vi "Main.vi"(11 "Module Admin":refnum<class "Delacor_lib_QMH_Module Admin.lvclass">) -> ()   [LabVIEW 2020, in "YP03-60CurrentSource_1.lvlib"]
doc: "This template is based off of the Queued Message Handler design pattern and the Queued Message Handler project template that ships with LabVIEW.\n\nThe main difference is that the queue is private to this module and communication between modules is performed via Broadcast and Request events.\n\nRequest events are wrapped in public API methods and are handled in the Event Handling Loop (EHL) of this VI. Any module can register for Broadcast events sent by this module. The EHL generates messages based on user interface actions.\n\nThe Message Handling Loop (MHL) processes messages generated by the EHL, or by other messages. The messages are string values, so new messages can be added easily to the Message Cases case structure in the MHL. Each message cluster can also provide an optional value for Message Data, which is a variant that can be converted to whatever message-specific data is required.\n_____\nBased on DQMH Project Template 6.0.0.91."
uses:
  YP03-60CurrentSource_1.lvlib
  <vilib>/Delacor/Delacor QMH/Libraries/Module Admin_class/Delacor_lib_QMH_Module Admin.lvclass
  CurrentSet-X Argument--cluster.ctl
  Module Data--cluster.ctl
  Stop Argument--cluster.ctl
  <vilib>/Delacor/Delacor QMH/Libraries/Message Queue_class/Delacor_lib_QMH_Message Queue.lvclass/Delacor_lib_QMH_Message Queue.ctl
  <vilib>/Delacor/Delacor QMH/Libraries/Module Admin_class/Delacor_lib_QMH_Module Admin.lvclass/Delacor_lib_QMH_Module Admin.ctl
  CurrentSet-Y Argument--cluster.ctl
  CurrentSet-Z Argument--cluster.ctl
  Output Argument--cluster.ctl
  <vilib>/Utility/miscctls.llb/LVPointTypeDef.ctl
  <vilib>/Delacor/Delacor QMH/Libraries/Message Queue_class/Delacor_lib_QMH_Enqueue Message (Single).vi
  <vilib>/Delacor/Delacor QMH/Libraries/Module Admin_class/Delacor_lib_QMH_Get External Launch.vi
  <vilib>/Utility/error.llb/Error Cluster From Error Code.vi
  <vilib>/ErrorRing/Error Ring.xnode
  <vilib>/Delacor/Delacor QMH/Libraries/Message Queue_class/Delacor_lib_QMH_Message Queue.lvclass
panel:
  in  "CurrentSet Argument":T1={"CurrentSet(A)"=0.0, "Cluster"={"VISA resource name"="COM6", "baud rate (9600)"=9600, "data bits (8)"=8, "parity (0:none)"=enum."None"}} {"Cluster"."data bits (8)" min=5 max=8 step=1; "CurrentSet(A)" min=-4.0 max=4.0 step=0.05}
  out "History:Entire Text":string="rev. 12 Tue, Feb 14, 2023 11:30:20 AM chenyu\r\n添加Request电流设置请求\n当外部调用该vi时，这个时间会被广播出去，被main函数生产结构接收到，进入从循环执行电流设置的vi\r\n"
  out "error out":errorcluster
  out "Status":string="Initial Message"
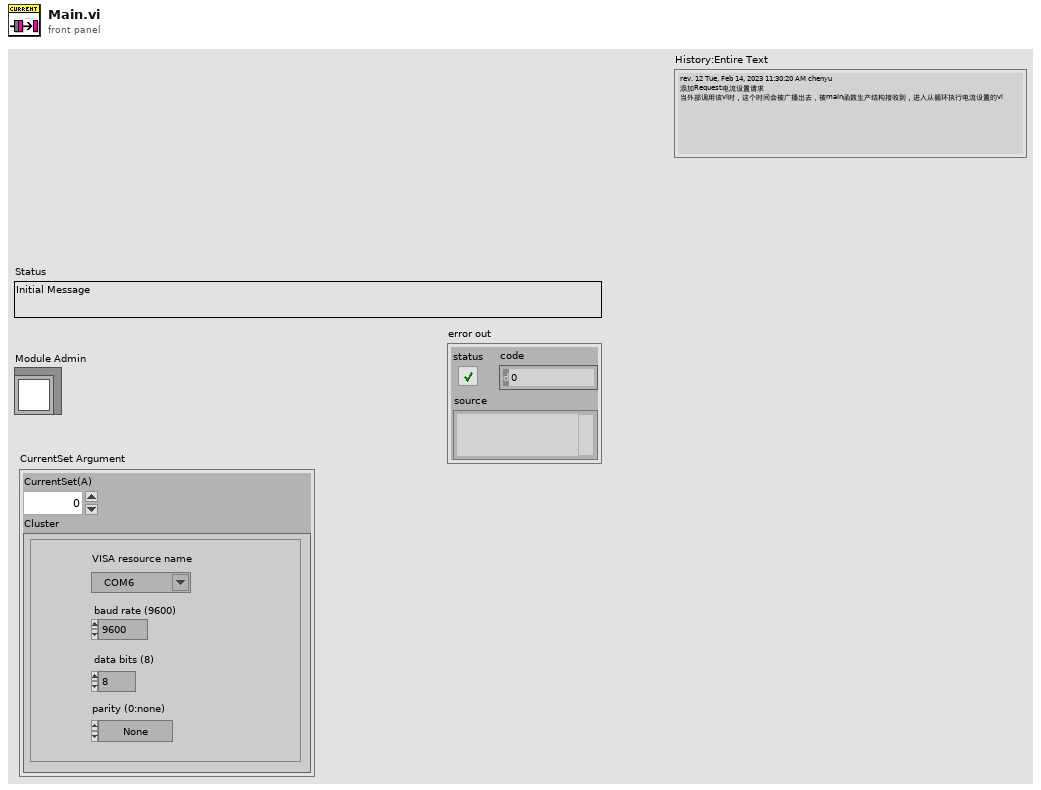
[diagram p1: front panel]
types:
  T1 = typedef "YP03-60CurrentSource_1.lvlib/CurrentSet-X Argument--cluster.ctl" = cluster{"CurrentSet(A)":dbl, "Cluster":cluster{"VISA resource name":refnum<visa-resource-name>, "baud rate (9600)":u32, "data bits (8)":u16, "parity (0:none)":enum16{"None", "Odd", "Even", "Mark", "Space"}}}
  T2 = typedef "YP03-60CurrentSource_1.lvlib/Request Events--cluster.ctl" = cluster{"Stop Module":refnum<user-event>, "Show Panel":refnum<user-event>, "Hide Panel":refnum<user-event>, "Get Module Execution Status":refnum<user-event>, "Show Diagram":refnum<user-event>, "CurrentSet-X":refnum<user-event>, "CurrentSet-Y":refnum<user-event>, "CurrentSet-Z":refnum<user-event>, "Output":refnum<user-event>}
  T3 = typedef "YP03-60CurrentSource_1.lvlib/Module Data--cluster.ctl" = cluster{"Status":string}
  T4 = enum32{"invalid lock state", "Not Locked", "Locked (No Password)", "Password-protected"}
  T5 = typedef "YP03-60CurrentSource_1.lvlib/Stop Argument--cluster.ctl" = cluster{"Origin":string, "Exit via Stop Module Req?":bool, "Wait for Module to stop?":bool}
  T6 = typedef "YP03-60CurrentSource_1.lvlib/CurrentSet-Y Argument--cluster.ctl" = cluster{"Cuurent-Y":dbl, "Cluster":cluster{"VISA resource name":refnum<visa-resource-name>, "baud rate (9600)":u32, "data bits (8)":u16, "parity (0:none)":enum16{"None", "Odd", "Even", "Mark", "Space"}}}
  T7 = typedef "YP03-60CurrentSource_1.lvlib/CurrentSet-Z Argument--cluster.ctl" = cluster{"Numeric":dbl, "Cluster":cluster{"VISA resource name":refnum<visa-resource-name>, "baud rate (9600)":u32, "data bits (8)":u16, "parity (0:none)":enum16{"None", "Odd", "Even", "Mark", "Space"}}}
  T8 = typedef "YP03-60CurrentSource_1.lvlib/Output Argument--cluster.ctl" = cluster{"Output":bool}
  T9 = typedef "LVPointTypeDef.ctl" = cluster{"Horizontal":i16, "Vertical":i16}
  T10 = enum32{"Invalid", "Standard", "Closed", "Hidden", "Minimized", "Maximized"}
  T11 = cluster{"VISA resource name":refnum<visa-resource-name>, "baud rate (9600)":u32, "data bits (8)":u16, "parity (0:none)":enum16{"None", "Odd", "Even", "Mark", "Space"}}
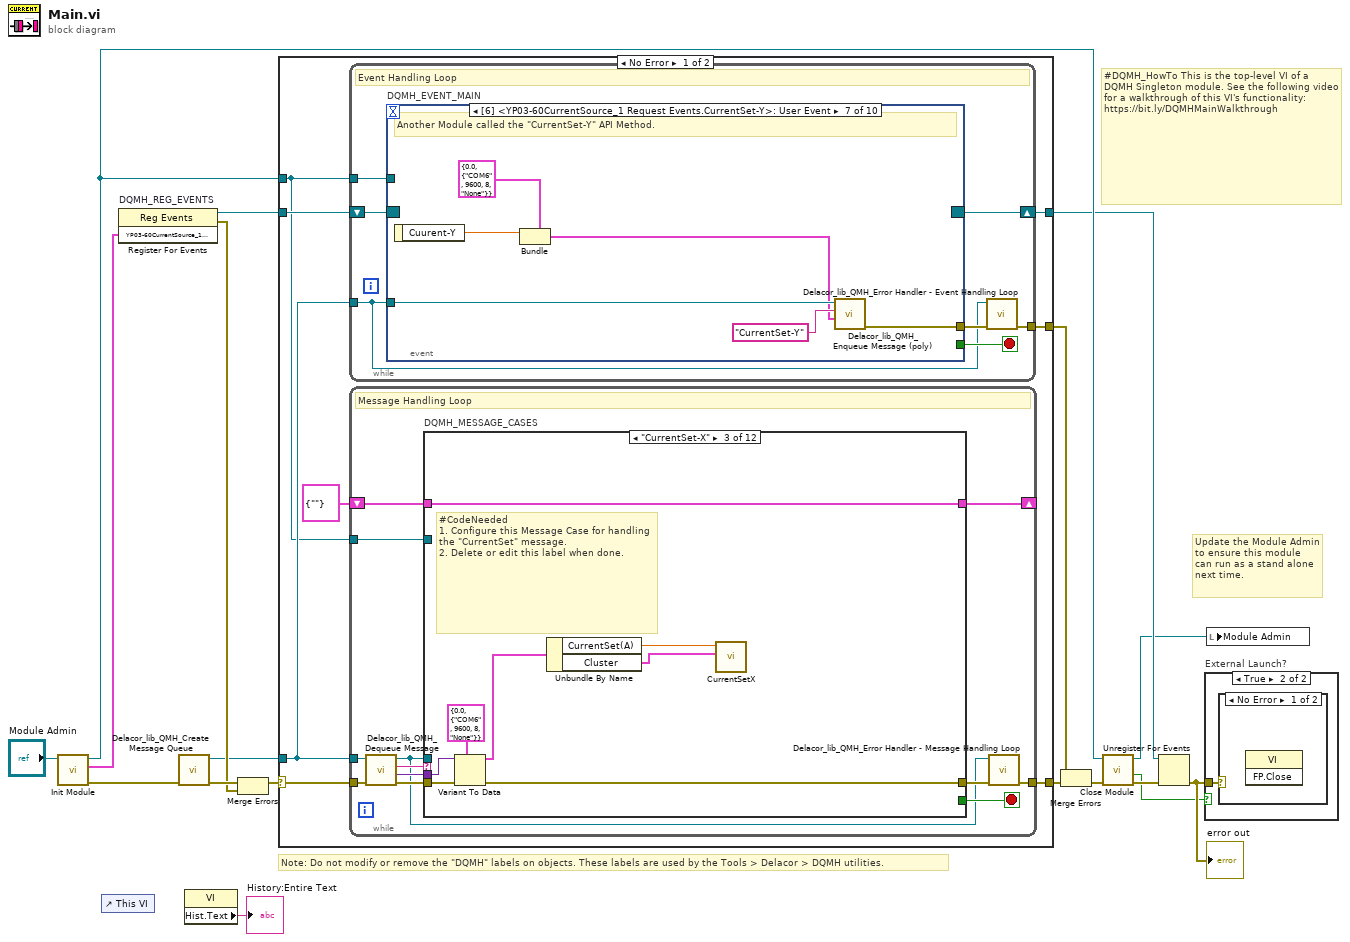
[diagram p0: block diagram]
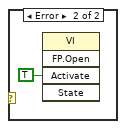
[diagram p3: hidden frame]
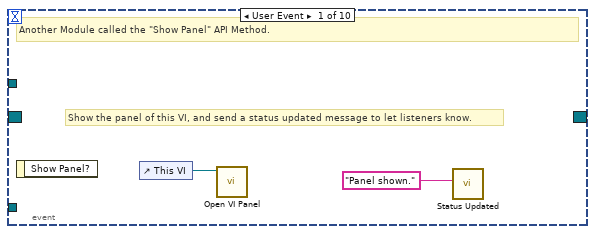
[diagram p4: hidden frame]
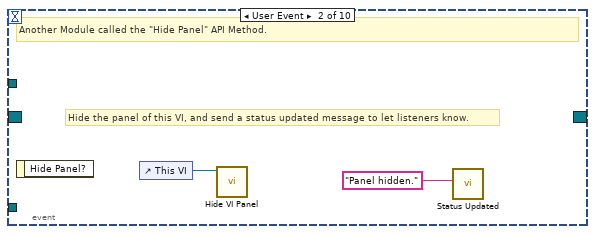
[diagram p5: hidden frame]
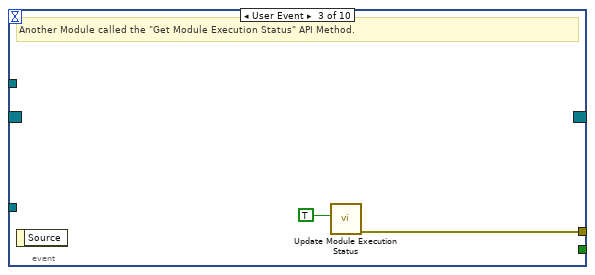
[diagram p6: hidden frame]
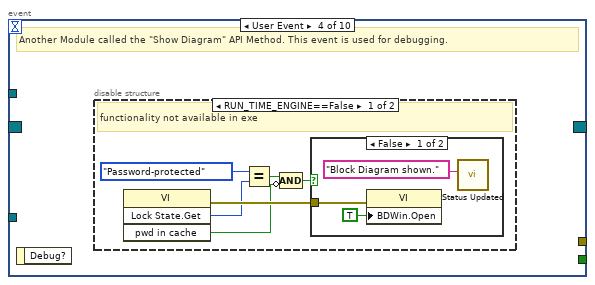
[diagram p7: hidden frame]
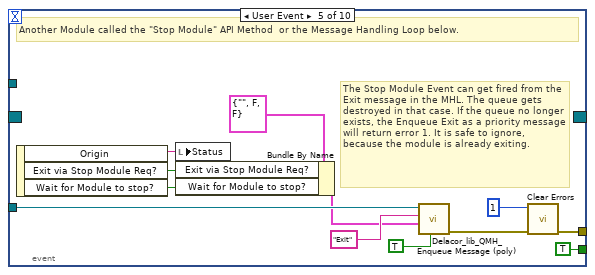
[diagram p10: hidden frame]
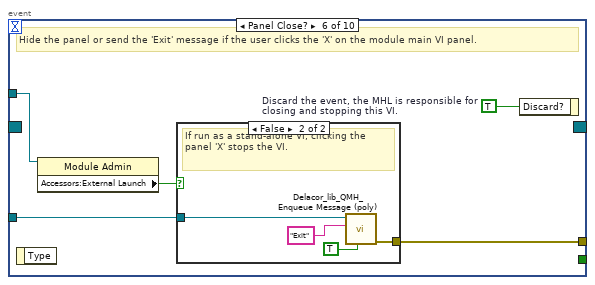
[diagram p11: hidden frame]
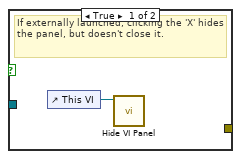
[diagram p12: hidden frame]
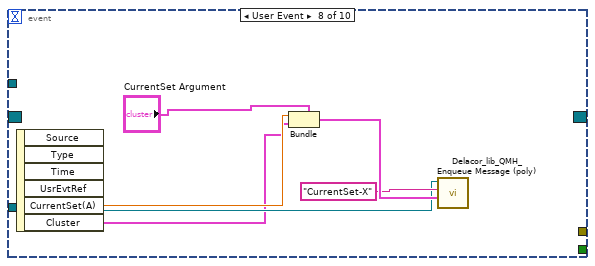
[diagram p13: hidden frame]
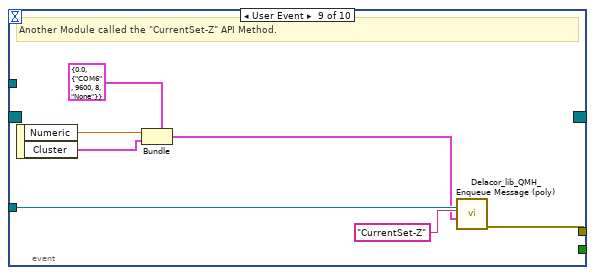
[diagram p14: hidden frame]
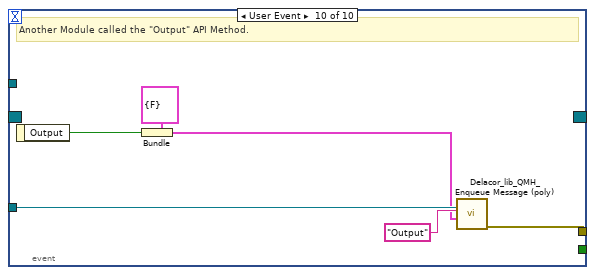
[diagram p15: hidden frame]
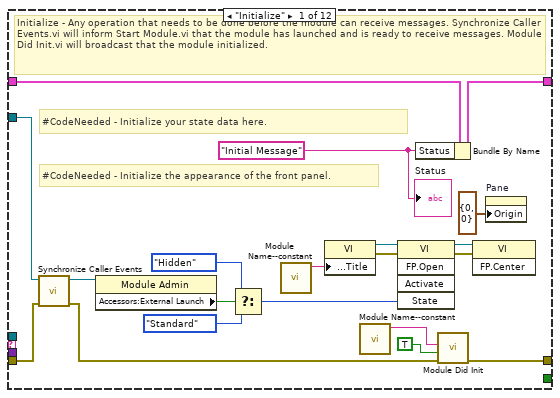
[diagram p16: hidden frame]
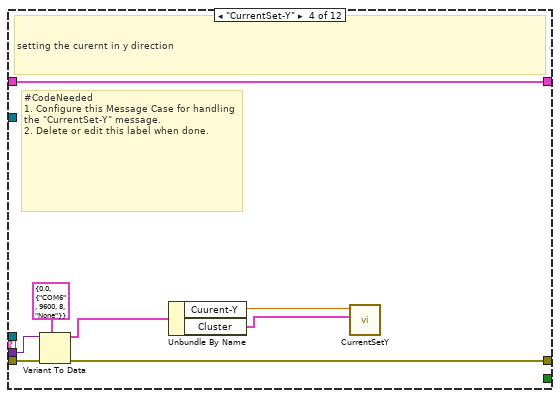
[diagram p18: hidden frame]
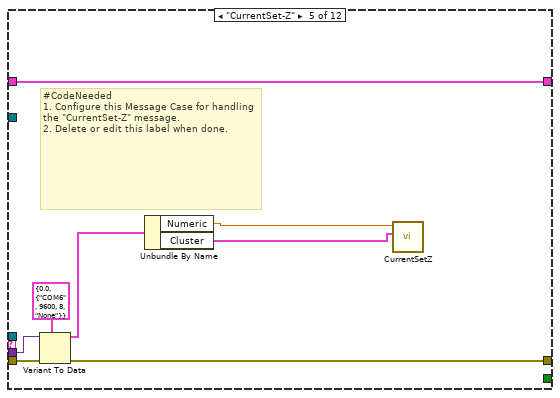
[diagram p19: hidden frame]
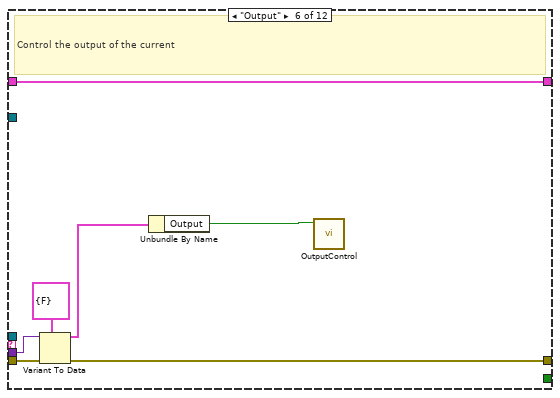
[diagram p20: hidden frame]
diagram:
  # "#DQMH_HowTo This is the top-level VI of a DQMH Singleton module. See the following video for a walkthrough of this VI's functionality: https://bit.ly/DQMHMainWalkthrough"
  # "Note: Do not modify or remove the \"DQMH\" labels on objects. These labels are used by the Tools > Delacor > DQMH utilities."
  # "Update the Module Admin to ensure this module can run as a stand alone next time."
  n1 = call "Init Module.vi"("Singleton Module Admin in"="Module Admin") -> ("error out"=w17:errorcluster, "YP03-60CurrentSource_1 Request Events"=w6:T2, "Singleton Module Admin out"=w9:refnum<class "Delacor_lib_QMH_Module Admin.lvclass">)  [unwired: 8 in]
  n2 = control-ref of="This VI"() -> ()  [unwired: 1 out]
  n3 = register-events "DQMH_REG_EVENTS"(w6) -> (reference out=w7:refnum<event-registration>, error out=w10:errorcluster)  [unwired: 2 in]
  n4 = call <vilib>:"Delacor_lib_QMH_Create Message Queue.vi"("error in"=w17) -> ("error out"=w12:errorcluster, "Message Queue"=w5:refnum<class "Delacor_lib_QMH_Message Queue.lvclass">)  [unwired: 9 in]
  n5 = property class="VI"() -> ("Hist.Text"=→"History:Entire Text":string)  [unwired: 2 in, 2 out]
  n6 = Merge Errors(w12, w10) -> (w11:errorcluster)
  n7 = case shown="No Error" w11 {
    selector: w11 -> [w24 w225]
    tunnel: [w26 w224] -> w18
    tunnel: [w23 w230] -> w8
    tunnel: w7 -> [w21 w230]
    tunnel: w5 -> [w20 w223]
    tunnel: [w25 _] -> w15
    tunnel: w9 -> [w19 w226]
    frame No Error {
      n8 = while {
        tunnel: w20 -> [w27]
        shift-right: [w30] -> w23
        shift-left: w21 -> [w31]
        tunnel: [w32] -> w25
        tunnel: w19 -> [w28]
        stop <- w29 stop-if-true
        # "Event Handling Loop"
        n9 = event "DQMH_EVENT_MAIN" shown="[6] <YP03-60CurrentSource_1 Request Events.CurrentSet-Y>: User Event" {
          selector: w31 -> [_ _ _ _ _ _ _ _ _ _]
          dyn-events: [_ _ _ _ _ _ _ _ _ _] -> w30
          timeout: _ -> [_ _ _ _ _ _ _ _ _ _]
          tunnel: [_ _ _ _ TRUE ("Discard?") _ _ _ _ _] -> w29
          tunnel: w27 -> [_ _ _ _ w56 w63 w76 w79 w89 w95]
          tunnel: [_ _ w39 _ w59 w65 w71 _ w84 w90] -> w33
          tunnel: w28 -> [_ _ _ _ _ w62 _ _ _ _]
          event User Event {
            # "Show the panel of this VI, and send a status updated message to let listeners know."
            # "Another Module called the \"Show Panel\" API Method."
            n10 = event-data() -> ()  [unwired: 1 in, 1 out]
            n11 = control-ref of="This VI"() -> (w35:refnum<vi>)
            n12 = call "Open VI Panel.vi"("VI"=w35) -> ()  [unwired: 10 in, 1 out]
            n13 = call "Status Updated.vi"("Status"="Panel shown." ("format string")) -> ()  [unwired: 10 in, 1 out]
          }
          event User Event {
            # "Hide the panel of this VI, and send a status updated message to let listeners know."
            # "Another Module called the \"Hide Panel\" API Method."
            n14 = event-data() -> ()  [unwired: 1 in, 1 out]
            n15 = control-ref of="This VI"() -> (w37:refnum<vi>)
            n16 = call "Hide VI Panel.vi"("VI"=w37) -> ()  [unwired: 10 in, 1 out]
            n17 = call "Status Updated.vi"("Status"="Panel hidden." ("format string")) -> ()  [unwired: 10 in, 1 out]
          }
          event User Event {
            # "Another Module called the \"Get Module Execution Status\" API Method."
            n18 = event-data() -> ()  [unwired: 1 in, 1 out]
            n19 = call "Update Module Execution Status.vi"("Running?"=TRUE) -> ("error out"=w39:errorcluster)  [unwired: 10 in]
          }
          event User Event {
            # "Another Module called the \"Show Diagram\" API Method. This event is used for debugging."
            n20 = event-data() -> ()  [unwired: 1 in, 1 out]
            n21 = disable-structure shown="RUN_TIME_ENGINE==False" {
              frame condition #0 (active) {
                # "functionality not available in exe"
                n22 = invoke class="VI" method="Lock State.Get"() -> (error out=w45:errorcluster, "Get Lock State"=w44:T4, "pwd in cache"=w41:bool)  [unwired: 4 in, 1 out]
                n23 = Equal?(x=T4."Password-protected", y=w44) -> (x = y?=w42:bool)
                n24 = Compound Arithmetic op=AND(w42, invert w41) -> (w40:bool)
                n25 = case shown="False" w40 {
                  tunnel: w45 -> [w48 _]
                  frame False {
                    n26 = property class="VI"(error in=w48, "BDWin.Open"=TRUE ("Block Diagram Window:Open")) -> ()  [unwired: 1 in, 2 out]
                    n27 = call "Status Updated.vi"("Status"="Block Diagram shown." ("format string")) -> ()  [unwired: 10 in, 1 out]
                  }
                  frame True {
                    # "Password-protected VI, and the password is not in the cache. Do not show the diagram."
                  }
                }
              }
              frame condition #1 {
              }
            }
          }
          event User Event {
            # "The Stop Module Event can get fired from the Exit message in the MHL. The queue gets destroyed in that case. If the queue no longer exists, the Enqueue Exit as a priority message will return error 1. It is safe to ignore, because the module is already exiting."
            # "Another Module called the \"Stop Module\" API Method  or the Message Handling Loop below."
            n28 = event-data() -> ("Origin"=w55:string, "Exit via Stop Module Req?"=w51:bool, "Wait for Module to stop?"=w50:bool)  [unwired: 1 in]
            n29 = local write "Status"(w55) -> ()
            n30 = Bundle By Name(cluster=T5 {"Origin"="", "Exit via Stop Module Req?"=FALSE, "Wait for Module to stop?"=FALSE} ("Stop Argument"), "Exit via Stop Module Req?"=w51, "Wait for Module to stop?"=w50) -> (w49:T5)
            n31 = call-poly <vilib>:"Delacor_lib_QMH_Enqueue Message (poly).vi"("Priority Message? (F)"=TRUE, "Message Data"=w49, "Message"="Exit", "Message Queue in"=w56) -> ("error out"=w60:errorcluster)  [unwired: 6 in, 1 out]
            n32 = call <vilib>:"Clear Errors.vi"("error in (no error)"=w60, "specific error code to clear (0: all)"=1) -> ("error out"=w59:errorcluster)  [unwired: 4 in, 1 out]
          }
          event Panel Close? {
            w64 = TRUE  # Discard the event, the MHL is responsible for closing and stopping this VI.
            # "Hide the panel or send the 'Exit' message if the user clicks the 'X' on the module main VI panel."
            n33 = event-data() -> ()  [unwired: 1 in, 1 out]
            n34 = property class="Module Admin"(reference=w62) -> ("Accessors:External Launch"=w61:bool)  [unwired: 1 in, 2 out]
            n35 = case shown="False" w61 {
              tunnel: w63 -> [_ w69]
              tunnel: [_ w70] -> w65
              frame True {
                # "If externally launched, clicking the 'X' hides the panel, but doesn't close it."
                n36 = control-ref of="This VI"() -> (w66:refnum<vi>)
                n37 = call "Hide VI Panel.vi"("VI"=w66) -> ()  [unwired: 10 in, 1 out]
              }
              frame False {
                # "If run as a stand-alone VI, clicking the panel 'X' stops the VI."
                n38 = call-poly <vilib>:"Delacor_lib_QMH_Enqueue Message (poly).vi"("Priority Message? (F)"=TRUE, "Message"="Exit", "Message Queue in"=w69) -> ("error out"=w70:errorcluster)  [unwired: 7 in, 1 out]
              }
            }
            n39 = event-data("Discard?"=w64) -> ()  [unwired: 1 in, 1 out]
          }
          event User Event {
            # "Another Module called the \"CurrentSet-Y\" API Method."
            n40 = event-data() -> ("Cuurent-Y"=w72:dbl)  [unwired: 1 in]
            n41 = Bundle(cluster=T6 {"Cuurent-Y"=0.0, "Cluster"={"VISA resource name"="COM6", "baud rate (9600)"=9600, "data bits (8)"=8, "parity (0:none)"=enum."None"}} ("CurrentSet-Y Argument"), "Cuurent-Y"=w72) -> (w73:T6)  [unwired: 1 in]
            n42 = call-poly <vilib>:"Delacor_lib_QMH_Enqueue Message (poly).vi"("Message Data"=w73, "Message"="CurrentSet-Y", "Message Queue in"=w76) -> ("error out"=w71:errorcluster)  [unwired: 7 in, 1 out]
          }
          event User Event {
            n43 = event-data() -> ("CurrentSet(A)"=w82:dbl, "Cluster"=w77:T11)  [unwired: 1 in, 4 out]
            n44 = Bundle(cluster="CurrentSet Argument", "CurrentSet(A)"=w82, "Cluster"=w77) -> (w81:T1)
            n45 = call-poly <vilib>:"Delacor_lib_QMH_Enqueue Message (poly).vi"("Message Data"=w81, "Message"="CurrentSet-X", "Message Queue in"=w79) -> ()  [unwired: 7 in, 2 out]
          }
          event User Event {
            # "Another Module called the \"CurrentSet-Z\" API Method."
            n46 = event-data() -> ("Numeric"=w85:dbl, "Cluster"=w83:T11)  [unwired: 1 in]
            n47 = Bundle(cluster=T7 {"Numeric"=0.0, "Cluster"={"VISA resource name"="COM6", "baud rate (9600)"=9600, "data bits (8)"=8, "parity (0:none)"=enum."None"}} ("CurrentSet-Z Argument"), "Numeric"=w85, "Cluster"=w83) -> (w86:T7)
            n48 = call-poly <vilib>:"Delacor_lib_QMH_Enqueue Message (poly).vi"("Message Data"=w86, "Message"="CurrentSet-Z", "Message Queue in"=w89) -> ("error out"=w84:errorcluster)  [unwired: 7 in, 1 out]
          }
          event User Event {
            # "Another Module called the \"Output\" API Method."
            n49 = event-data() -> ("Output"=w91:bool)  [unwired: 1 in]
            n50 = Bundle(cluster=T8 {"Output"=FALSE} ("Output Argument"), "Output"=w91) -> (w92:T8)
            n51 = call-poly <vilib>:"Delacor_lib_QMH_Enqueue Message (poly).vi"("Message Data"=w92, "Message"="Output", "Message Queue in"=w95) -> ("error out"=w90:errorcluster)  [unwired: 7 in, 1 out]
          }
        }
        n52 = call-dynamic "Delacor_lib_QMH_Error Handler - Event Handling Loop.vi"("error in"=w33, "Message Queue in"=w27) -> ("dup error in"=w32:errorcluster)  [unwired: 8 in, 1 out]
      }
      n53 = while {
        tunnel: w20 -> [w98]
        shift-right: [w102] -> _
        shift-left: T3 {"Status"=""} ("Data Cluster") -> [w103]
        tunnel: w24 -> [w106]
        tunnel: [w104] -> w26
        tunnel: w19 -> [w96]
        stop <- w101 stop-if-true
        # "Message Handling Loop"
        n54 = call-dynamic "Delacor_lib_QMH_Dequeue Message.vi"("error in"=w106, "Message Queue in"=w98) -> ("error out"=w105:errorcluster, "Message Data"=w99:variant, "Message"=w100:string, "Message Queue out"=w97:refnum<class "Delacor_lib_QMH_Message Queue.lvclass">)  [unwired: 6 in]
        n55 = case "DQMH_MESSAGE_CASES" shown="\"CurrentSet-X\"" w100 {
          selector: w100 -> [_ _ _ _ _ _ _ _ _ _ _ w210]
          tunnel: w97 -> [_ _ _ _ _ _ _ _ _ w180 w202 _]
          tunnel: w105 -> [w125 w129 w137 w145 w153 w160 w163 w165 w170 w187 w208 w212]
          tunnel: [w123 w129 w135 w143 w151 w158 w162 w165 w169 w183 w205 w213] -> w107
          tunnel: w103 -> [w114 w128 w136 w144 w152 w159 w161 w164 w167 w182 w201 w211]
          tunnel: [w113 w128 w136 w144 w152 w159 w161 w164 w167 w182 w201 w211] -> w102
          tunnel: [_ _ _ _ _ _ _ _ _ _ w200 _] -> w101
          tunnel: w99 -> [_ _ w134 w142 w150 w157 _ _ _ w181 w199 _]
          tunnel: w96 -> [w115 _ _ _ _ _ _ _ _ w179 w194 _]
          frame "Initialize" {
            w109 = "Initial Message" ("Initial Message")
            # "#CodeNeeded - Initialize the appearance of the front panel."
            # "#CodeNeeded - Initialize your state data here."
            # "Initialize - Any operation that needs to be done before the module can receive messages. Synchronize Caller Events.vi will inform Start Module.vi that the module has launched and is ready to receive messages. Module Did Init.vi will broadcast that the module initialized."
            n56 = call "Synchronize Caller Events.vi"("error in (no error)"=w125, "Singleton Module Admin in"=w115) -> ("error out"=w124:errorcluster, "Singleton Module Admin out"=w110:refnum<class "Delacor_lib_QMH_Module Admin.lvclass">)  [unwired: 8 in]
            n57 = property class="Module Admin"(reference=w110) -> ("Accessors:External Launch"=w119:bool)  [unwired: 1 in, 2 out]
            n58 = Select(t=T10."Hidden" ("State"), s=w119, f=T10."Standard" ("State")) -> (s? t:f=w116:T10)
            n59 = call "Module Name--constant.vi"() -> ("Module Name"=w122:string)  [unwired: 11 in]
            n60 = property class="VI"("Front Panel.Title"=w122) -> (reference out=w121:refnum<vi>, error out=w127:errorcluster)  [unwired: 2 in]
            n61 = call "Module Name--constant.vi"() -> ("Module Name"=w111:string)  [unwired: 11 in]
            n62 = invoke class="VI" method="FP.Open"(reference=w121, error in=w127, "State"=w116) -> (reference out=w120:refnum<vi>, error out=w126:errorcluster)  [unwired: 2 in, 3 out]
            n63 = Bundle By Name(cluster=w114, "Status"=w109) -> (w113:T3)
            n64 = call "Module Did Init.vi"("error in (no error)"=w124, "Initialized?"=TRUE, "Origin"=w111) -> ("error out"=w123:errorcluster)  [unwired: 8 in]
            n65 = invoke class="VI" method="FP.Center"(reference=w120, error in=w126) -> ()  [unwired: 1 in, 3 out]
            n66 = property on="Pane" class="Pane"("Origin"=T9 {"Horizontal"=0, "Vertical"=0}) -> ()  [unwired: 2 in, 2 out]
            "Status" <- w109
          }
          frame "---Module Specific---" {
            # "Separator -- The following cases handle messages specific to this Module."
          }
          frame "CurrentSet-X" {
            # "#CodeNeeded\n1. Configure this Message Case for handling the \"CurrentSet\" message.\n2. Delete or edit this label when done."
            n67 = Variant To Data(error in=w137, type=T1 {"CurrentSet(A)"=0.0, "Cluster"={"VISA resource name"="COM6", "baud rate (9600)"=9600, "data bits (8)"=8, "parity (0:none)"=enum."None"}} ("CurrentSet Argument"), Variant=w134) -> (data=w132:T1, error out=w135:errorcluster)
            n68 = Unbundle By Name(w132) -> ("CurrentSet(A)"=w131:dbl, "Cluster"=w130:T11)
            n69 = call "CurrentSetX.vi"("Cluster"=w130, "电流设置"=w131) -> ()  [unwired: 10 in]
          }
          frame "CurrentSet-Y" {
            # "#CodeNeeded\n1. Configure this Message Case for handling the \"CurrentSet-Y\" message.\n2. Delete or edit this label when done."
            # "setting the curernt in y direction"
            n70 = Variant To Data(error in=w145, type=T6 {"Cuurent-Y"=0.0, "Cluster"={"VISA resource name"="COM6", "baud rate (9600)"=9600, "data bits (8)"=8, "parity (0:none)"=enum."None"}} ("CurrentSet-Y Argument"), Variant=w142) -> (data=w140:T6, error out=w143:errorcluster)
            n71 = Unbundle By Name(w140) -> ("Cuurent-Y"=w139:dbl, "Cluster"=w138:T11)
            n72 = call "CurrentSetY.vi"("Cluster"=w138, "电流设置"=w139) -> ()  [unwired: 10 in]
          }
          frame "CurrentSet-Z" {
            # "#CodeNeeded\n1. Configure this Message Case for handling the \"CurrentSet-Z\" message.\n2. Delete or edit this label when done."
            n73 = Variant To Data(error in=w153, type=T7 {"Numeric"=0.0, "Cluster"={"VISA resource name"="COM6", "baud rate (9600)"=9600, "data bits (8)"=8, "parity (0:none)"=enum."None"}} ("CurrentSet-Z Argument"), Variant=w150) -> (data=w148:T7, error out=w151:errorcluster)
            n74 = Unbundle By Name(w148) -> ("Numeric"=w147:dbl, "Cluster"=w146:T11)
            n75 = call "CurrentSetZ.vi"("Cluster"=w146, "电流设置"=w147) -> ()  [unwired: 9 in, 1 out]
          }
          frame "Output" {
            # "Control the output of the current"
            n76 = Variant To Data(error in=w160, type=T8 {"Output"=FALSE} ("Output Argument"), Variant=w157) -> (data=w155:T8, error out=w158:errorcluster)
            n77 = Unbundle By Name(w155) -> ("Output"=w154:bool)
            n78 = call "OutputControl.vi"("输出控制"=w154) -> ()  [unwired: 11 in]
          }
          frame "---Copy This Frame---" {
            # "Duplicate this frame when creating new messages.  Change this comment in the duplicated frame to describe this message."
            n79 = Merge Errors(w163) -> (w162:errorcluster)
          }
          frame "---Exit and Error Handling---" {
            # "Separator - The following cases handle errors and exit messages."
          }
          frame "Simulate MHL Error" {
            # "#DQMH_HowTo The 'Simulate MHL Error' button  illustrates how the MHL handles errors. This event is instructional in nature and can be removed."
            # "Simulate an error occurring at the MHL"
            n80 = call "Module Name--constant.vi"() -> ("Module Name"=w166:string)  [unwired: 11 in]
            n81 = xnode "Error Ring"("parameter 0"=w166) -> ("error out"=w168:errorcluster)
            n82 = Merge Errors(w170, w168) -> (w169:errorcluster)
          }
          frame "Error" {
            # "#CodeRecommended - If you ever change the name of this \"Error\" message, you'll need to update the name in the Check Loop Error.vi as well."
            # "#CodeRecommended - If the module is running in standalone mode (External Launch = FALSE), this code will pop up an error dialog and call the 'Exit' message if an error occurs. Add more fine-grained error handling here."
            # "Error - Check the error message data and respond accordingly. This message is sent by the \"Error Handler\" VIs at the end of each loop in this application."
            n83 = property class="Module Admin"(reference=w179) -> ("Accessors:External Launch"=w178:bool)  [unwired: 1 in, 2 out]
            n84 = Variant To Data(error in=w187, type=errorcluster {"status"=FALSE, "code"=0, "source"=""} ("error constant"), Variant=w181) -> (data=w188:errorcluster, error out=w185:errorcluster)
            n85 = call "Error Reported.vi"("Error"=w188) -> ()  [unwired: 10 in, 1 out]
            n86 = case shown="False" w178 {
              tunnel: [w193 _] -> w184
              tunnel: w180 -> [w191 _]
              tunnel: w188 -> [w192 _]
              frame False {
                # "If the module is running standalone, then pop up an error dialog and call the \"Exit\" message."
                n87 = call <vilib>:"Simple Error Handler.vi"("error in (no error)"=w192) -> ()  [unwired: 4 in, 5 out]
                n88 = call-poly <vilib>:"Delacor_lib_QMH_Enqueue Message (poly).vi"("Priority Message? (F)"=TRUE, "Message"="Exit", "Message Queue in"=w191) -> ("error out"=w193:errorcluster)  [unwired: 7 in, 1 out]
              }
              frame True {
                # "If the module was launched externally, calling the Error Reported broadcast VI is the only action performed by the \"Error\" message. The module's caller can then process the error appropriately."
              }
            }
            n89 = Merge Errors(w185, w184) -> (w183:errorcluster)
            n90 = local write "error out"(w183) -> ()
          }
          frame "Exit" {
            w198 = 91  # 91: not all Exit messages will have an argument
            w200 = TRUE  # Stop the VI
            # "Release the message queue reference"
            # "#CodeNeeded - Add any required cleanup code here"
            # "Exit - Exit the application."
            n91 = Variant To Data(error in=w208, type=T5 {"Origin"="", "Exit via Stop Module Req?"=FALSE, "Wait for Module to stop?"=FALSE} ("Stop Argument"), Variant=w199) -> (data=w196:T5, error out=w204:errorcluster)
            n92 = call <vilib>:"Clear Errors.vi"("error in (no error)"=w204, "specific error code to clear (0: all)"=w198) -> ("error out"=w207:errorcluster)  [unwired: 4 in, 1 out]
            n93 = control-ref of="This VI"() -> (w195:refnum<vi>)
            n94 = call-dynamic "Delacor_lib_QMH_Release Message Queue.vi"("error in"=w207, "Message Queue"=w202) -> ("error out"=w206:errorcluster)  [unwired: 9 in]
            n95 = call "Handle Exit.vi"("Stop Argument"=w196, "Admin in"=w194, "VI reference"=w195) -> ("error out"=w203:errorcluster)  [unwired: 7 in, 1 out]
            n96 = Merge Errors(w206, w203) -> (w205:errorcluster)
          }
          frame Default {
            # "'Default' case only runs if there is a message that isn't defined in any of the other cases.  Output a programming error."
            n97 = call "Module Name--constant.vi"() -> ("Module Name"=w209:string)  [unwired: 11 in]
            n98 = xnode "Error Ring"("parameter 0"=w210, "parameter 1"=w209) -> ("error out"=w214:errorcluster)
            n99 = Merge Errors(w212, w214) -> (w213:errorcluster)
          }
        }
        n100 = call-dynamic "Delacor_lib_QMH_Error Handler - Message Handling Loop.vi"("error in"=w107, "Message Queue in"=w97) -> ("dup error in"=w104:errorcluster)  [unwired: 8 in, 1 out]
      }
    }
    frame Error {
      # "Synchronize Caller Events.vi will inform Start Module.vi that the module has launched and will let the code calling Start Module.vi register for broadcasts and would permit the caller receive the broadcast that an error occurred at launch time."
      n101 = call-dynamic "Delacor_lib_QMH_Release Message Queue.vi"("error in"=w225, "Message Queue"=w223) -> ("error out"=w224:errorcluster)  [unwired: 9 in]
      n102 = call "Synchronize Caller Events.vi"("Singleton Module Admin in"=w226) -> ("error out"=w231:errorcluster)  [unwired: 9 in, 1 out]
      n103 = call "Module Name--constant.vi"() -> ("Module Name"=w229:string)  [unwired: 11 in]
      n104 = Format Into String(format string="An error occurred during initialization. %s is no longer running.", w229) -> (resulting string=w227:string)  [unwired: 2 in, 1 out]
      n105 = Merge Errors(w224, w231) -> (w232:errorcluster)
      n106 = call "Error Reported.vi"("Additional Information"=w227, "Error"=w232) -> ()  [unwired: 9 in, 1 out]
    }
  }
  n107 = Merge Errors(w15, w18) -> (w14:errorcluster)
  n108 = call "Close Module.vi"("error in (no error)"=w14, "Module Admin in"=w9) -> ("error out"=w16:errorcluster, "External Launch"=w2:bool, "Module Admin out"=w3:refnum<class "Delacor_lib_QMH_Module Admin.lvclass">)  [unwired: 7 in]
  n109 = Unregister For Events(event registration refnum=w8, error in=w16) -> (error out=w13:errorcluster)
  "error out" <- w13
  n110 = case "External Launch?" shown="True" w2 {
    tunnel: w13 -> [_ w233]
    frame False {
    }
    frame True {
      n111 = case shown="No Error" w233 {
        frame No Error {
          n112 = invoke class="VI" method="FP.Close"() -> ()  [unwired: 3 in, 3 out]
        }
        frame Error {
          n113 = invoke class="VI" method="FP.Open"("Activate"=TRUE ("Activate?")) -> ()  [unwired: 4 in, 5 out]
        }
      }
    }
  }
  n114 = local write "Module Admin"(w3) -> ()
